vi "Calibration_Load.vi"(11 "Data in":T2={"L16 Linear Actuator"="", "XE 1000 Pump"="", "Camera1"="", "Camera2"="", "Camera1_IMG"=refnum, "Camera2_IMG"=refnum, "Img_Capt"=FALSE, "Actuator"=FALSE, "Pump"=FALSE, "Cam 1"=FALSE, "Cam 2"=FALSE, "Empty_Refill"=FALSE, "Crop"=FALSE, "Light intensity"=100, "Exposure Time"=1000.0, "Sample Name"="Test Sample", "Operator"="MRJ", "Calibration 1"=path "C:/Users/au540322/Desktop/IHS_Project/images/Debris/Debris_0/Debris_0_2019_06_01-23-32-49-686.PNG", "Calibration 2"=path "C:/Users/au540322/Desktop/IHS_Project/images/Debris/Debris_0/Debris_0_2019_06_01-23-32-49-686.PNG", "Framerate"=1, "Timeout Sample"=200, "Collection date"="", "Sample size threshold"=1, "Empty start"=1, "Command"="MRJ", "Calibration Image 1"=refnum, "Calibration Image 2"=refnum, "Original Image 1"=refnum, "Original Image 2"=refnum, "Processing Image 1"=refnum, "Processing Image 2"=refnum, "Object Image 1"=refnum, "Object Image 2"=refnum, "Cam 1 - save queue"=refnum, "Cam 2 - save queue"=refnum, "Station"="", "Species Name"="", "Other Notes"="", "Aperture"=enum."Item 0", "Image Process Queue Size"=500, "Image Save Queue Size"=500, "Overload threshold"=500, "Max Framerate"=100, "Blue Plane Image"=refnum, "Subtract Image"=refnum, "Binary Image 1"=refnum, "ROI mask allocation"=refnum, "Rectangle 1"={"Left"=0, "Top"=0, "Right"=0, "Bottom"=0, "Rotation"=0.0}, "Rectangle 2"={"Left"=0, "Top"=0, "Right"=0, "Bottom"=0, "Rotation"=0.0}, "Binary Image 2"=refnum, "Detection Region %"=0.0, "Cam 1 queue"=refnum, "Cam 2 queue"=refnum, "Detect image 1"=refnum, "Detect image 2"=refnum, "Detect 1"=path "C:/Users/au540322/Desktop/IHS_Project/images/Debris/Debris_0/Debris_0_2019_06_01-23-32-49-686.PNG", "Detect 2"=path "C:/Users/au540322/Desktop/IHS_Project/images/Debris/Debris_0/Debris_0_2019_06_01-23-32-49-686.PNG", "Max large object threshold"=0, "Open(T)/Close(F)"=FALSE} {"Rectangle 2"."Rotation" format="%.2f"; "Rectangle 2"."Left" scale=0.0..1024.0; "Rectangle 2"."Right" scale=0.0..1024.0; "Rectangle 1"."Rotation" format="%.2f"; "Rectangle 1"."Left" scale=0.0..1024.0; "Rectangle 1"."Right" scale=0.0..1024.0; "Max Framerate" min=1; "Overload threshold" min=1; "Image Save Queue Size" min=1; "Image Process Queue Size" min=1; "Empty start" min=1; "Sample size threshold" min=1; "Framerate" min=1; "Light intensity" scale=0.0..100.0}) -> (0 "Next State":T1=enum."Wait for Event", 2 "Calibration error?":bool, 3 "Data out":T2={"L16 Linear Actuator"="", "XE 1000 Pump"="", "Camera1"="", "Camera2"="", "Camera1_IMG"=refnum, "Camera2_IMG"=refnum, "Img_Capt"=FALSE, "Actuator"=FALSE, "Pump"=FALSE, "Cam 1"=FALSE, "Cam 2"=FALSE, "Empty_Refill"=FALSE, "Crop"=FALSE, "Light intensity"=100, "Exposure Time"=1000.0, "Sample Name"="Test Sample", "Operator"="MRJ", "Calibration 1"=path "C:/Users/au540322/Desktop/IHS_Project/images/Debris/Debris_0/Debris_0_2019_06_01-23-32-49-686.PNG", "Calibration 2"=path "C:/Users/au540322/Desktop/IHS_Project/images/Debris/Debris_0/Debris_0_2019_06_01-23-32-49-686.PNG", "Framerate"=100, "Timeout Sample"=200, "Collection date"="", "Sample size threshold"=500, "Empty start"=1, "Command"="", "Calibration Image 1"=refnum, "Calibration Image 2"=refnum, "Original Image 1"=refnum, "Original Image 2"=refnum, "Processing Image 1"=refnum, "Processing Image 2"=refnum, "Object Image 1"=refnum, "Object Image 2"=refnum, "Cam 1 - save queue"=refnum, "Cam 2 - save queue"=refnum, "Station"="", "Species Name"="", "Other Notes"="", "Aperture"=enum."Item 0", "Image Process Queue Size"=500, "Image Save Queue Size"=500, "Overload threshold"=500, "Max Framerate"=100, "Blue Plane Image"=refnum, "Subtract Image"=refnum, "Binary Image 1"=refnum, "ROI mask allocation"=refnum, "Rectangle 1"={"Left"=0, "Top"=0, "Right"=0, "Bottom"=0, "Rotation"=0.0}, "Rectangle 2"={"Left"=0, "Top"=0, "Right"=0, "Bottom"=0, "Rotation"=0.0}, "Binary Image 2"=refnum, "Detection Region %"=0.0, "Cam 1 queue"=refnum, "Cam 2 queue"=refnum, "Detect image 1"=refnum, "Detect image 2"=refnum, "Detect 1"=path "C:/Users/au540322/Desktop/IHS_Project/images/Debris/Debris_0/Debris_0_2019_06_01-23-32-49-686.PNG", "Detect 2"=path "C:/Users/au540322/Desktop/IHS_Project/images/Debris/Debris_0/Debris_0_2019_06_01-23-32-49-686.PNG", "Max large object threshold"=0, "Open(T)/Close(F)"=FALSE} {"Rectangle 2"."Rotation" format="%.2f"; "Rectangle 2"."Left" scale=0.0..1024.0; "Rectangle 2"."Right" scale=0.0..1024.0; "Rectangle 1"."Rotation" format="%.2f"; "Rectangle 1"."Left" scale=0.0..1024.0; "Rectangle 1"."Right" scale=0.0..1024.0; "Max Framerate" min=1; "Overload threshold" min=1; "Image Save Queue Size" min=1; "Image Process Queue Size" min=1; "Empty start" min=1; "Sample size threshold" min=1; "Framerate" min=1; "Light intensity" scale=0.0..100.0})   [LabVIEW 2019]
uses:
  controls/Data.ctl
  <vilib>/userdefined/High Color/IMAQdx.ctl
  <vilib>/vision/Image Controls.llb/IMAQ Image.ctl
  controls/State.ctl
  <vilib>/vision/NI_Vision_Development_Module.lvlib
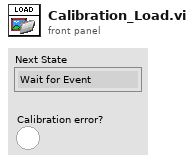
[diagram p1: front panel]
types:
  T1 = typedef "State.ctl" = enum16{"Initialize", "Wait for Event", "Position", "Valve Signal", "Extra Flush", "Valve Cycle", "Valve Open", "Valve Close", "Pump Command", "Pump Cycle", "Empty System", "Start System", "Connect Systems", "Start Image Capture", "Stop Image Capture", "Calibration Pictures", "Empty and Refill", "Change Light Intensity", "Reconnect", "Exit"}
  T2 = typedef "Data.ctl" = cluster{"L16 Linear Actuator":refnum<visa-resource-name>, "XE 1000 Pump":refnum<visa-resource-name>, "Camera1":T3, "Camera2":T3, "Camera1_IMG":T4, "Camera2_IMG":T4, "Img_Capt":bool, "Actuator":bool, "Pump":bool, "Cam 1":bool, "Cam 2":bool, "Empty_Refill":bool, "Crop":bool, "Light intensity":i32, "Exposure Time":dbl, "Sample Name":string, "Operator":string, "Calibration 1":path, "Calibration 2":path, "Framerate":i32, "Timeout Sample":i32, "Collection date":string, "Sample size threshold":i32, "Empty start":u32, "Command":string, "Calibration Image 1":T4, "Calibration Image 2":T4, "Original Image 1":T4, "Original Image 2":T4, "Processing Image 1":T4, "Processing Image 2":T4, "Object Image 1":T4, "Object Image 2":T4, "Cam 1 - save queue":refnum<queue>, "Cam 2 - save queue":refnum<queue>, "Station":string, "Species Name":string, "Other Notes":string, "Aperture":enum32{"Item 0", "Item 1", "Item 2", "Item 3"}, "Image Process Queue Size":i32, "Image Save Queue Size":i32, "Overload threshold":i32, "Max Framerate":i32, "Blue Plane Image":T4, "Subtract Image":T4, "Binary Image 1":T4, "ROI mask allocation":T4, "Rectangle 1":T5, "Rectangle 2":T5, "Binary Image 2":T4, "Detection Region %":dbl, "Cam 1 queue":refnum<queue>, "Cam 2 queue":refnum<queue>, "Detect image 1":T4, "Detect image 2":T4, "Detect 1":path, "Detect 2":path, "Max large object threshold":i32, "Open(T)/Close(F)":bool}
  T3 = typedef "IMAQdx.ctl" = refnum<k21>
  T4 = typedef "IMAQ Image.ctl" = refnum<image>
  T5 = typedef "IMAQ Rectangle" = cluster{"Left":i32, "Top":i32, "Right":i32, "Bottom":i32, "Rotation":dbl}
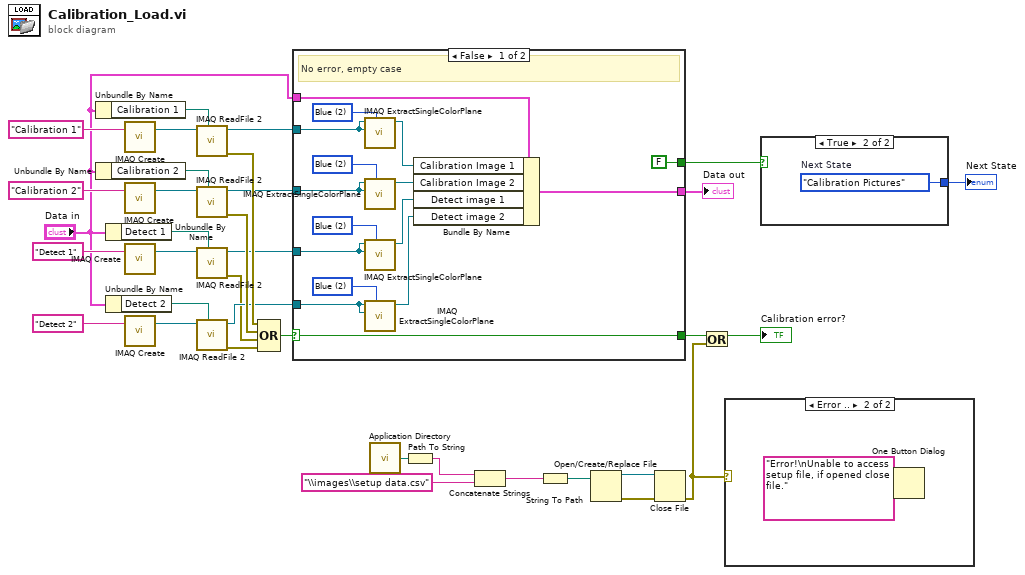
[diagram p0: block diagram]
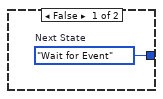
[diagram p3: hidden frame]
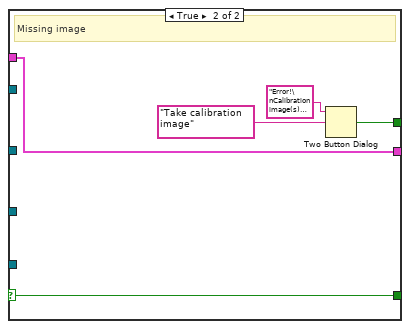
[diagram p4: hidden frame]
diagram:
  n1 = Unbundle By Name("Data in") -> ("Calibration 1"=w33:path)
  n2 = Unbundle By Name("Data in") -> ("Calibration 2"=w30:path)
  n3 = Unbundle By Name("Data in") -> ("Detect 1"=w12:path)
  n4 = Unbundle By Name("Data in") -> ("Detect 2"=w10:path)
  n5 = call "IMAQ Create"("Image Name"="Calibration 1") -> ("New Image"=w34:T4)  [unwired: 3 in, 2 out]
  n6 = call "IMAQ Create"("Image Name"="Calibration 2") -> ("New Image"=w31:T4)  [unwired: 3 in, 2 out]
  n7 = call "IMAQ Create"("Image Name"="Detect 1") -> ("New Image"=w18:T4)  [unwired: 3 in, 2 out]
  n8 = call "IMAQ Create"("Image Name"="Detect 2") -> ("New Image"=w16:T4)  [unwired: 3 in, 2 out]
  n9 = call "IMAQ ReadFile 2"("File Path"=w33, "Image"=w34) -> ("error out"=w27:errorcluster, "Image Out"=w21:T4)  [unwired: 5 in, 3 out]
  n10 = call "IMAQ ReadFile 2"("File Path"=w30, "Image"=w31) -> ("error out"=w28:errorcluster, "Image Out"=w22:T4)  [unwired: 5 in, 3 out]
  n11 = call "IMAQ ReadFile 2"("File Path"=w12, "Image"=w18) -> ("error out"=w14:errorcluster, "Image Out"=w17:T4)  [unwired: 5 in, 3 out]
  n12 = call "IMAQ ReadFile 2"("File Path"=w10, "Image"=w16) -> ("error out"=w13:errorcluster, "Image Out"=w15:T4)  [unwired: 5 in, 3 out]
  n13 = Compound Arithmetic op=OR(w27, w28, w14, w13) -> (w29:bool)
  n14 = case shown="False" w29 {
    selector: w29 -> [w48 w52]
    tunnel: "Data in" -> [w51 w54]
    tunnel: [w50 w54] -> w26
    tunnel: [FALSE ("T button?") w53] -> w25
    tunnel: [w48 w52] -> w24
    tunnel: w22 -> [w46 _]
    tunnel: w21 -> [w44 _]
    tunnel: w17 -> [w39 _]
    tunnel: w15 -> [w38 _]
    frame False {
      w40 = 2 items=["Red", "Green", "Blue", "Hue", "Saturation", "Luminance", "Value", "Intensity"] ("Color Plane")
      w41 = 2 items=["Red", "Green", "Blue", "Hue", "Saturation", "Luminance", "Value", "Intensity"] ("Color Plane")
      w45 = 2 items=["Red", "Green", "Blue", "Hue", "Saturation", "Luminance", "Value", "Intensity"] ("Color Plane")
      w47 = 2 items=["Red", "Green", "Blue", "Hue", "Saturation", "Luminance", "Value", "Intensity"] ("Color Plane")
      # "No error, empty case"
      n15 = call "IMAQ ExtractSingleColorPlane"("Color Plane"=w45, "Image Dst"=w44, "Image Src"=w44) -> ("Image Dst Out"=w42:T4)  [unwired: 1 in, 7 out]
      n16 = call "IMAQ ExtractSingleColorPlane"("Color Plane"=w47, "Image Dst"=w46, "Image Src"=w46) -> ("Image Dst Out"=w43:T4)  [unwired: 1 in, 7 out]
      n17 = call "IMAQ ExtractSingleColorPlane"("Color Plane"=w41, "Image Dst"=w39, "Image Src"=w39) -> ("Image Dst Out"=w37:T4)  [unwired: 1 in, 7 out]
      n18 = call "IMAQ ExtractSingleColorPlane"("Color Plane"=w40, "Image Dst"=w38, "Image Src"=w38) -> ("Image Dst Out"=w36:T4)  [unwired: 1 in, 7 out]
      n19 = Bundle By Name(cluster=w51, "Calibration Image 1"=w42, "Calibration Image 2"=w43, "Detect image 1"=w37, "Detect image 2"=w36) -> (w50:T2)
    }
    frame True {
      # "Missing image"
      n20 = Two Button Dialog(message="Error!\nCalibration image(s) missing!", 2:"Take calibration image" ("T button name (\"OK\")")) -> (T button?=w53:bool)  [unwired: 1 in]
    }
  }
  "Data out" <- w26
  n21 = call <vilib>:"Application Directory.vi"() -> ("Application Directory"=w9:path)
  n22 = Path To String(path=w9) -> (string=w8:string)
  n23 = Concatenate Strings(w8, "\\images\\setup data.csv") -> (w6:string)
  n24 = String To Path(string=w6) -> (path=w5:path)
  n25 = Open/Create/Replace File(file path (use dialog)=w5) -> (refnum out=w4:refnum<file>, error out=w3:errorcluster)  [unwired: 5 in, 1 out]
  n26 = Close File(refnum=w4, error in=w3) -> (error out=w1:errorcluster)  [unwired: 1 out]
  n27 = Or(x=w24, y=w1) -> (x .or. y?=→"Calibration error?":bool)
  n28 = case shown="Error .." w1 {
    frame No Error {
    }
    frame Error {
      n29 = One Button Dialog(message="Error!\nUnable to access setup file, if opened close file.") -> ()  [unwired: 1 in, 1 out]
    }
  }
  n30 = case shown="True" w25 {
    tunnel: [w58 w59] -> w23
    frame False {
      w58 = State."Wait for Event"  # Next State
    }
    frame True {
      w59 = State."Calibration Pictures"  # Next State
    }
  }
  "Next State" <- w23
